vi "ReadPersonData.vi"(0 "reference in":refnum<class "MyTestClass.lvclass">, 5 "error in (no error)":errorcluster) -> (14 "reference out":refnum<class "MyTestClass.lvclass">, 15 "Name":string, 16 "Address":string, 17 "City":string, 19 "error out":errorcluster)   [LabVIEW 2020, in "MyTestClass.lvclass"]
uses:
  MyTestClass.lvclass
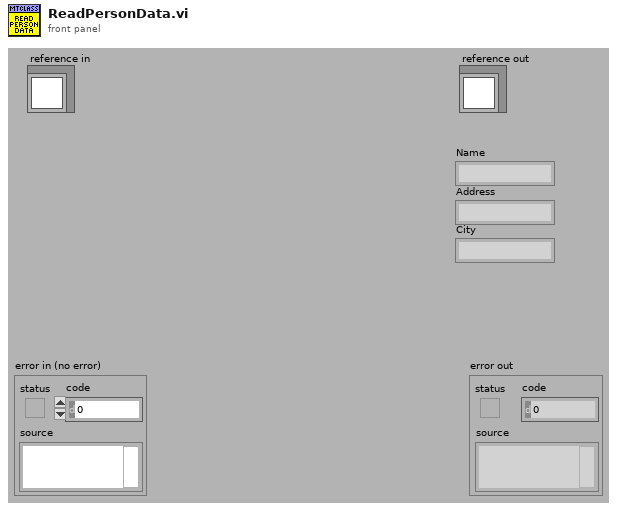
[diagram p1: front panel]
types:
  T1 = typedef "MyTestClass.lvclass/ObjectAttributes.ctl" = cluster{"Name":string, "Address":string, "City":string}
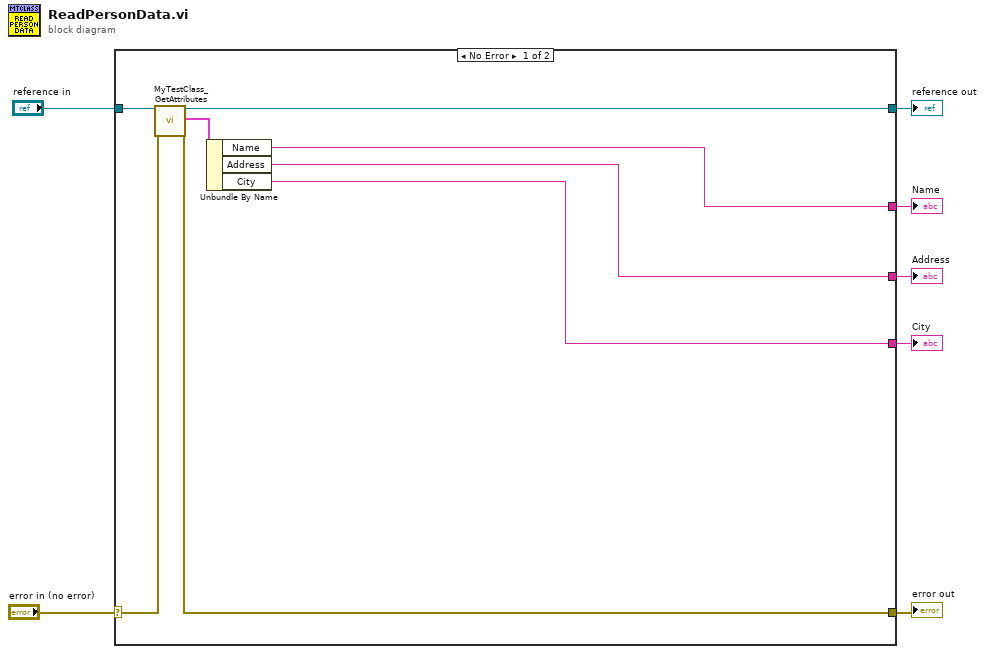
[diagram p0: block diagram]
diagram:
  n1 = case shown="No Error" "error in (no error)" {
    selector: "error in (no error)" -> [w15 w17]
    tunnel: [w13 w17] -> w6
    tunnel: [w11 w16] -> w4
    tunnel: "reference in" -> [w12 w16]
    tunnel: [w10 _] -> w3
    tunnel: [w9 _] -> w2
    tunnel: [w8 _] -> w1
    frame No Error {
      n2 = call "MyTestClass_GetAttributes.vi"("reference in"=w12, "error in (no error)"=w15) -> ("reference out"=w11:refnum<class "MyTestClass.lvclass">, "attributes"=w14:T1, "error out"=w13:errorcluster)  [unwired: 14 in, 1 out]
      n3 = Unbundle By Name(w14) -> ("Name"=w10:string, "Address"=w9:string, "City"=w8:string)
    }
    frame Error {
    }
  }
  "error out" <- w6
  "reference out" <- w4
  "City" <- w1
  "Address" <- w2
  "Name" <- w3
